vi "GlobComm.vi"() -> ()   [LabVIEW 2014]
panel:
  in  "Timeout":i32=4000
  in  "max bytes/read":i32=2500
  in  "Number of datagrams to read":u32=5000 format="%0d"
  in  "initialized":bool
  in  "commandmessageType":u32=17476 format="%x"
  in  "commanditems":u8=4
  in  "Port Receive":u16=5678
  in  "invert_send":bool=TRUE
  in  "host":string="192.168.1.18"
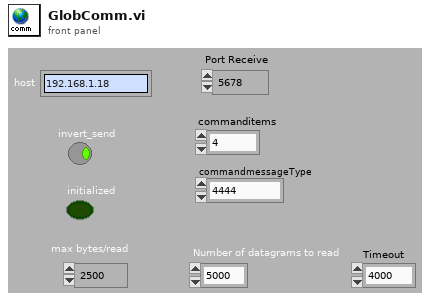
[diagram p1: front panel]
diagram:
